vi "calculateSpectraTest.vi"(7 "Reset?":bool, 8 "ErrorIn":errorcluster, 9 "AnalysisSettings":T1={"Fault Thresholds"={"Parameters labels"=[], "Parameters thresholds"=[], "Freqs and thresholds"=[], "Orders and thresholds"=[]}, "Analysis series name"="Analiza", "Save data analysis?"=TRUE, "F-Band Size"=20, "OrderAnalysis?"=TRUE, "Accelerometer"=enum."MMA7351", "fs [Hz]"=4000.0, "Pulse per revolution"=1, "FFT-Parameters"={"averaging mode"=enum."No averaging", "weighting mode"=enum."Linear", "number of averages"=0}, "O-WindowPowerSpectrum"=0, "O-SpectrumAveraging"=enum."No averaging", "O-MaxOrder"=0.0, "O-Resolution"=0.0, "O-BandSize"=0.0, "FrameLength [s]"=1.0, "Aq.FrameLength [ms]"=0, "FilterOrder"=0, "Sensitivity [V/g]"=[]}, 10 "Tacho signal In":waveform(dbl), 11 "AccelerationDataIn":waveform(dbl)[](array[waveform])) -> (0 "ErrorOut":errorcluster, 1 "Rotational speed [RPM]":dbl format="%0.2f", 2 "AccelerationDataFrames":T12, 3 "Tacho signal out":waveform(dbl), 4 "order power spectra":T11(array[cluster]) {"order 0" format="%.2p"; "delta order" format="%.2p"; "magnitude" format="%.2f"}, 5 "AccelerationDataOut":waveform(dbl)[](array[waveform]), 6 "spectrum info":T5[](array[typedef]) {"x-axis units" items=["Time (s)"=0, "Frequency-CB (Hz)"=1, "Frequency-CPB (Hz)"=1248, "Frequency-Arbitrary (Hz)"=2357, "Quefrency (s)"=2, "Revolutions (rev)"=3, "Order"=4, "Speed (RPM)"=11, "Speed (rad/s)"=21, "Index"=65535]; "weighting filter" items=["Linear", "A-weighting", "B-weighting", "C-weighting", "ITU-R 468-4", "Dolby", "CCITT", "C-message", "Wb", "Wc", "Wd", "We", "Wf", "Wh", "Wj", "Wk", "Wm", "AES17 20 kHz lowpass", "AES17 40 kHz lowpass", "AES17 20 kHz highpass", "AES17 40 kHz highpass"]; "dB reference [EU]" format="%.2f"; "engineering units" items=["custom..."=0, "V"=1, "A"=21, "C"=30, "pC"=31, "s"=32, "-"=29, "Pa"=2, "N"=20, "g"=3, "m/s^2"=4, "m/s"=5, "m"=6, "mm/s"=12, "mm"=13, "micron/s"=14, "micron"=15, "in/s^2"=7, "in/s"=8, "in"=9, "mil/s"=10, "mil"=11, "rad/s^2"=16, "rad/s"=17, "rad"=18, "deg/s^2"=26, "deg/s"=27, "deg"=28, "RPM"=22, "cycle/s^2"=23, "Hz"=24, "cycle"=25, "strain"=19]; "spectral info"."window" items=["None "=0, "Hanning"=1, "Hamming"=2, "Blackman-Harris"=3, "Exact Blackman"=4, "Blackman"=5, "Flat Top"=6, "4 Term B-Harris "=7, "7 Term B-Harris"=8, "Low Sidelobe"=9, "Force - Exponential"=10, "Gaussian"=62]})   [LabVIEW 2019]
uses:
  MobileAnalyzer/mainVIs/analyzeAccelerationDataVIs/AccelerationDataFrames.ctl
  <vilib>/addons/_NISVFA/_Shared subVIs/Controls/svc_Spectrum Info.ctl
  <vilib>/addons/_NISVFA/_Shared subVIs/Controls/svc_X-Axis Units.ctl
  <vilib>/addons/_NISVFA/_Shared subVIs/Controls/svc_Spectrum Type.ctl
  <vilib>/addons/_NISVFA/_Shared subVIs/Controls/svc_Engineering Units Text Ring.ctl
  <vilib>/addons/_NISVFA/_Shared subVIs/Controls/svc_Weighting Filter Text Ring.ctl
  <vilib>/addons/_NISVFA/_Shared subVIs/Controls/svc_Complimentary Spectrum Units.ctl
  VibrationDiagnosisDesktopApp/mainVIs/DialogsVIs/AnalysisSettings.ctl
  MobileAnalyzer/mainVIs/analyzeAccelerationDataVIs/calculateFaultIndicatorsVIs/Thresholds.ctl
  MobileAnalyzer/mainVIs/analyzeAccelerationDataVIs/calculateFaultIndicatorsVIs/FaultParameter.ctl
  MobileAnalyzer/mainVIs/aquireAccelerationDataVIs/Accelerometer.ctl
  <vilib>/Analysis/baseanly.llb/Mean (DBL).vi
  <vilib>/measure/maspectr.llb/FFT Spectrum (Mag-Phase) for N Chan.vi
  <vilib>/addons/Sound and Vibration/Order Analysis/Tach Process/OAT Analog Tacho Process (1 Tacho).vi
  <vilib>/addons/Sound and Vibration/Order Analysis/Resample Order Tracking/OAT Convert to Even Angle Signal (N Channels).vi
  <vilib>/addons/Sound and Vibration/Order Analysis/Utility/OAT Output Triggered Even Angle Signal (N Channels).vi
  <vilib>/addons/Sound and Vibration/Order Analysis/Resample Order Tracking/OAT Order Power Spectrum (N Channels).vi
  <vilib>/addons/Sound and Vibration/Order Analysis/Tach Process/SoundVib_TachProcess.lvlib
  <vilib>/addons/Sound and Vibration/Order Analysis/Resample Order Tracking/SoundVib_OrderTracking.lvlib
  <vilib>/Waveform/WDTOps.llb/WDT Waveform Duration DBL.vi
  <vilib>/Waveform/WDTOps.llb/WDT Get Waveform Subset DBL.vi
  <vilib>/Analysis/NI_AALBase.lvlib
  <vilib>/measure/NI_MAPro.lvlib
  <vilib>/addons/Sound and Vibration/Order Analysis/Utility/SoundVib_OAUtility.lvlib
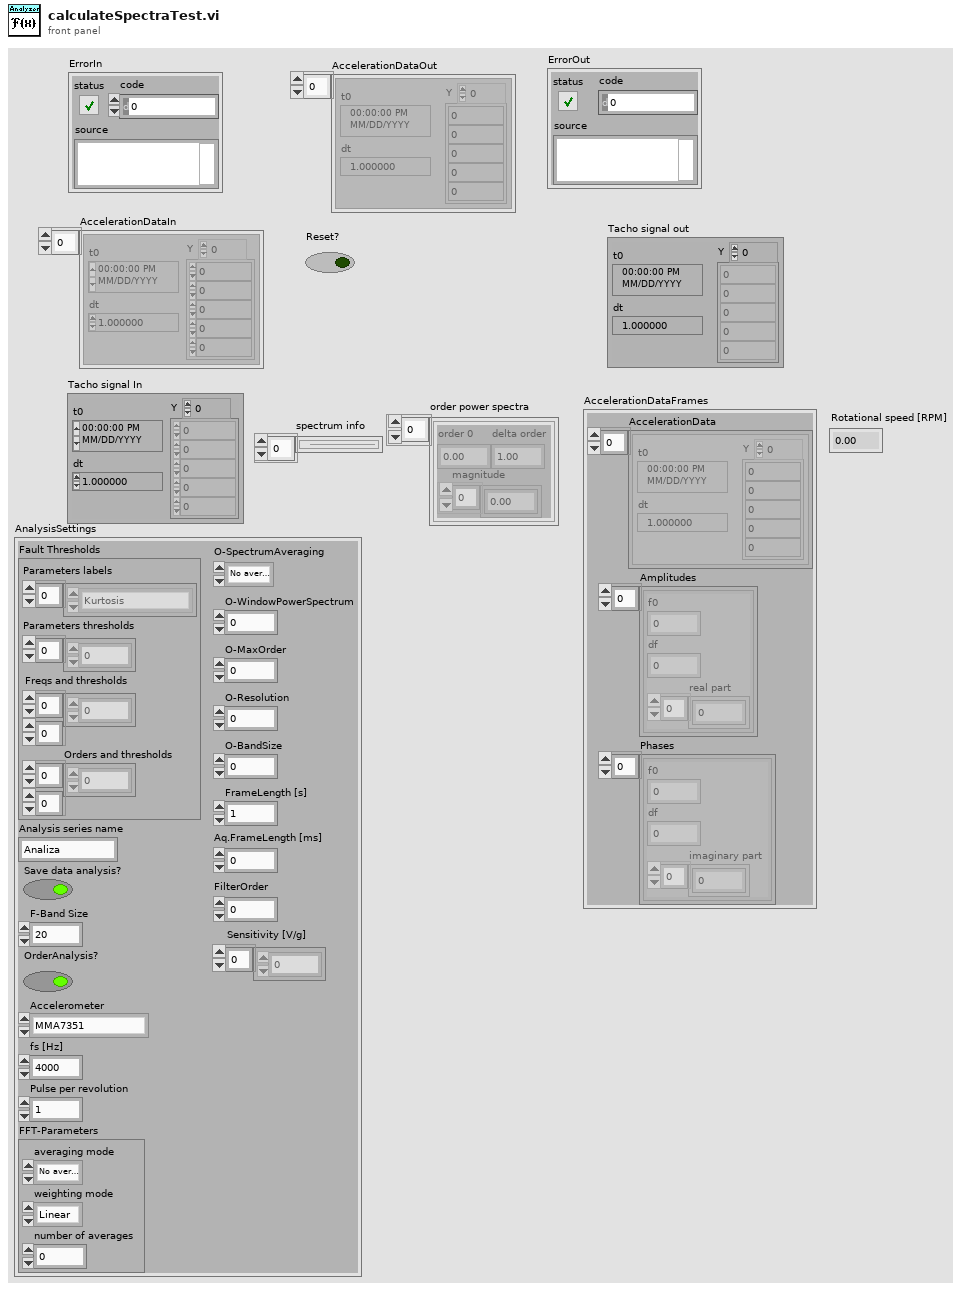
[diagram p1: front panel]
types:
  T1 = typedef "AnalysisSettings.ctl" = cluster{"Fault Thresholds":T2, "Analysis series name":string, "Save data analysis?":bool, "F-Band Size":i32, "OrderAnalysis?":bool, "Accelerometer":T4, "fs [Hz]":dbl, "Pulse per revolution":u16, "FFT-Parameters":cluster{"averaging mode":enum16{"No averaging", "Vector averaging", "RMS averaging", "Peak hold"}, "weighting mode":enum16{"Linear", "Exponential"}, "number of averages":u32}, "O-WindowPowerSpectrum":u32, "O-SpectrumAveraging":enum16{"No averaging", "Vector averaging", "RMS averaging", "Peak hold"}, "O-MaxOrder":dbl, "O-Resolution":dbl, "O-BandSize":dbl, "FrameLength [s]":dbl, "Aq.FrameLength [ms]":i64, "FilterOrder":i32, "Sensitivity [V/g]":dbl[]}
  T2 = typedef "Thresholds.ctl" = cluster{"Parameters labels":T3[], "Parameters thresholds":dbl[], "Freqs and thresholds":dbl[][], "Orders and thresholds":dbl[][]}
  T3 = typedef "FaultParameter.ctl" = enum16{"Kurtosis", "RMS", "Crest factor"}
  T4 = typedef "Accelerometer.ctl" = enum16{"None", "MPU6050", "MMA7351"}
  T5 = typedef "svc_Spectrum Info.ctl" = cluster{"channel name":string, "description":string, "x-axis units":T6, "spectral info":cluster{"spectrum type":T7, "linear/dB":enum16{"linear", "dB"}, "window":u16, "window size":i32, "FFT size":i32}, "engineering units":T8, "custom label":string, "dB reference [EU]":dbl, "peak units":enum16{"rms", "peak", "peak-peak"}, "weighting filter":T9, "spectral density?":bool, "unit label":string, "spectrum skewed?":bool, "complimentary spectrum units":T10}
  T6 = typedef "svc_X-Axis Units.ctl" = u16
  T7 = typedef "svc_Spectrum Type.ctl" = enum16{"FFT Spectrum [complex]", "Amplitude [Magnitude]", "Power [Magnitude^2]", "Cross Spectrum [complex]", "Frequency Response [Complex]"}
  T8 = typedef "svc_Engineering Units Text Ring.ctl" = u16
  T9 = typedef "svc_Weighting Filter Text Ring.ctl" = u16
  T10 = typedef "svc_Complimentary Spectrum Units.ctl" = enum16{"none", "radians", "degrees", "cycles", "imaginary"}
  T11 = cluster{"order 0":dbl, "delta order":dbl, "magnitude":dbl[]}[]
  T12 = typedef "AccelerationDataFrames.ctl" = cluster{"AccelerationData":waveform(dbl)[], "Amplitudes":cluster{"f0":dbl, "df":dbl, "real part":dbl[]}[], "Phases":cluster{"f0":dbl, "df":dbl, "imaginary part":dbl[]}[]}
  T13 = cluster{"averaging mode":enum16{"No averaging", "Vector averaging", "RMS averaging", "Peak hold"}, "weighting mode":enum16{"Linear", "Exponential"}, "number of averages":u32, "linear mode":enum16{"One shot", "Auto restart"}}
  T14 = cluster{"averaging mode":enum16{"No averaging", "Vector averaging", "RMS averaging", "Peak hold"}, "weighting mode":enum16{"Linear", "Exponential"}, "number of averages":u32}
  T15 = enum16{"No averaging", "Vector averaging", "RMS averaging", "Peak hold"}
  T16 = typedef "SoundVib_TachProcess.lvlib/speed profile.ctl" = cluster{"time [s]":dbl[], "speed [RPM]":dbl[]}
  T17 = typedef "svc_Resampled Channel Info.ctl" = cluster{"channel name":string, "description":string, " channel info":T18}
  T18 = typedef "svc_Channel Info.ctl" = cluster{"sensor sensitivity":dbl, "engineering units":T8, "dB reference":dbl, "custom label":string, "weighting filter":T9, "pregain":dbl}
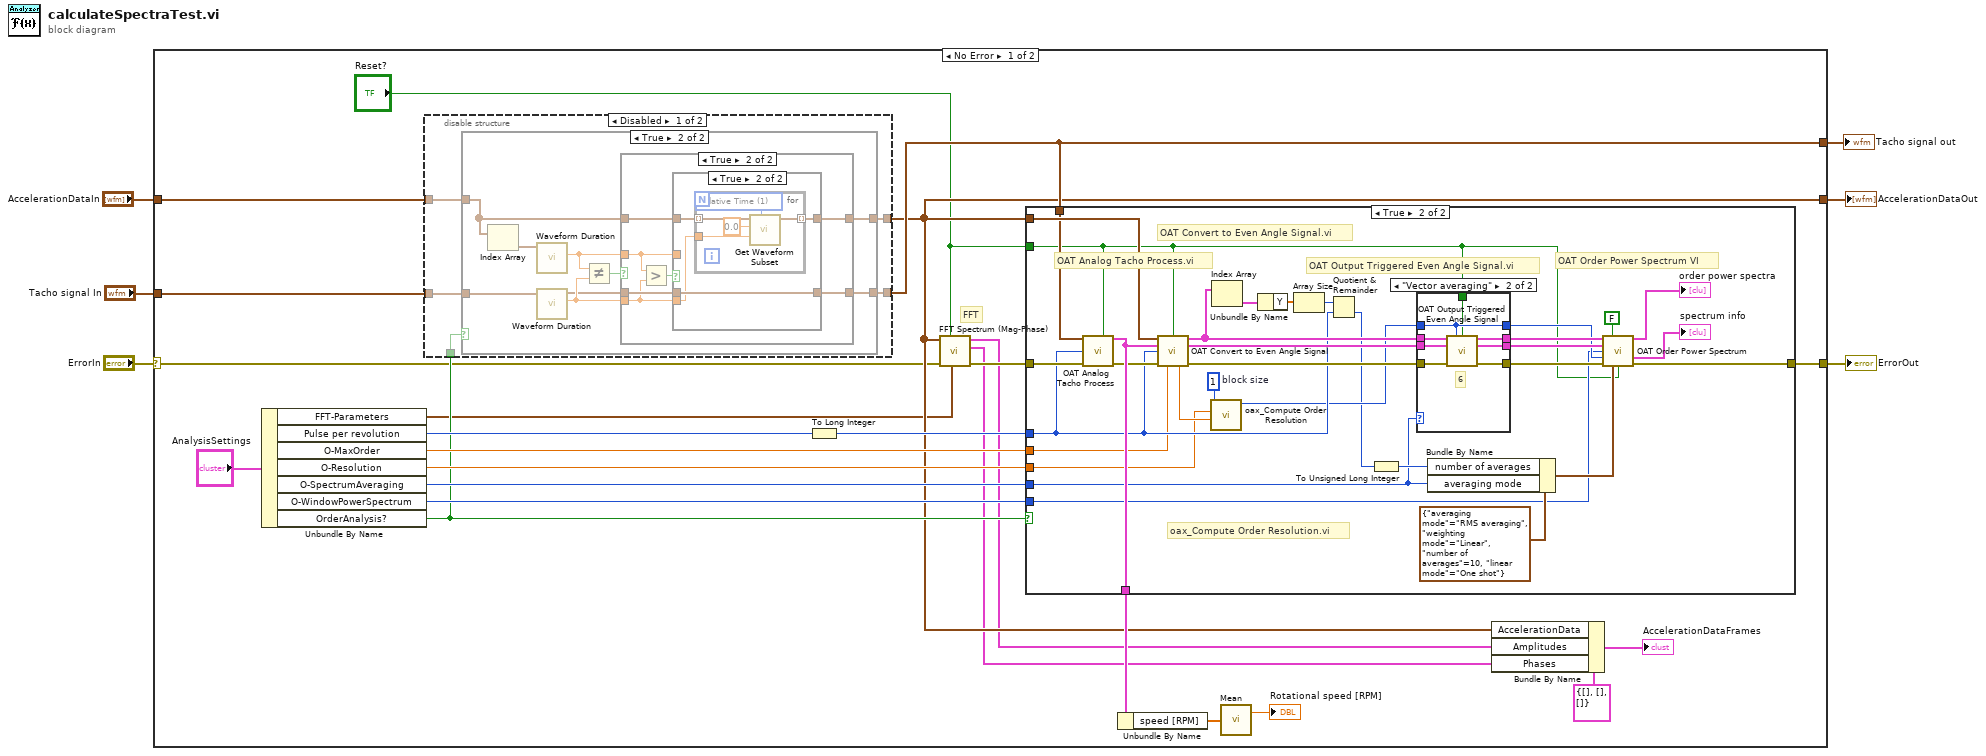
[diagram p0: block diagram]
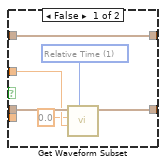
[diagram p4: hidden frame]
diagram:
  n1 = case shown="No Error" "ErrorIn" {
    selector: "ErrorIn" -> [w11 w120]
    tunnel: [w24 w120] -> w6
    tunnel: "AccelerationDataIn" -> [w28 w119]
    tunnel: [w13 w119] -> w3
    tunnel: "Tacho signal In" -> [w27 w118]
    tunnel: [w23 w118] -> w1
    frame No Error {
      # "FFT"
      n2 = Unbundle By Name("AnalysisSettings") -> ("FFT-Parameters"=w10:T14, "Pulse per revolution"=w19:u16, "O-MaxOrder"=w18:dbl, "O-Resolution"=w17:dbl, "O-SpectrumAveraging"=w16:T15, "O-WindowPowerSpectrum"=w15:u32, "OrderAnalysis?"=w14:bool)
      n3 = disable-structure shown="Disabled" {
        disable-tunnel: w28 -> [w35 w72]
        disable-tunnel: w27 -> [w34 w71]
        disable-tunnel: [w33 w71] -> w23
        disable-tunnel: w14 -> [w32 _]
        disable-tunnel: [w31 w72] -> w13
        frame Disabled {
          n4 = case shown="True" w32 {
            tunnel: w35 -> [w37 w41]
            tunnel: w34 -> [w36 w40]
            tunnel: [w37 w39] -> w31
            tunnel: [w36 w38] -> w33
            frame False {
            }
            frame True {
              n5 = Index Array(array=w41) -> (element=w42:waveform(dbl))  [unwired: 1 in]
              n6 = call-poly <vilib>:"Waveform Duration.vi"("waveform in"=w42) -> ("duration"=w45:dbl)  [unwired: 8 in, 2 out]
              n7 = call-poly <vilib>:"Waveform Duration.vi"("waveform in"=w40) -> ("duration"=w46:dbl, "waveform out"=w44:waveform(dbl))  [unwired: 8 in, 1 out]
              n8 = Not Equal?(x=w45, y=w46) -> (x != y?=w43:bool)
              n9 = case shown="True" w43 {
                tunnel: w41 -> [w48 w53]
                tunnel: w44 -> [w47 w54]
                tunnel: [w48 w49] -> w39
                tunnel: [w47 w50] -> w38
                tunnel: w45 -> [_ w52]
                tunnel: w46 -> [_ w51]
                frame False {
                }
                frame True {
                  n10 = Greater?(x=w52, y=w51) -> (0:w55:bool)
                  n11 = case shown="True" w55 {
                    tunnel: w54 -> [w61 w65]
                    tunnel: w53 -> [w58 w64]
                    tunnel: w52 -> [w60 _]
                    tunnel: w51 -> [_ w63]
                    tunnel: [w59 w65] -> w50
                    tunnel: [w58 w62] -> w49
                    frame False {
                      w56 = u16 1 items=["Samples", "Relative Time"] ("start/duration format")
                      n12 = call-poly <vilib>:"Get Waveform Subset.vi"("start/duration format"=w56, "duration"=w60, "start samples/time"=0.0, "waveform in"=w61) -> ("waveform out"=w59:waveform(dbl))  [unwired: 2 in, 3 out]
                    }
                    frame True {
                      n13 = for {
                        tunnel: w64 -> [w70] mode=indexing
                        tunnel: w63 -> [w69]
                        tunnel: [w68] -> w62 mode=indexing
                        w66 = u16 1 items=["Samples", "Relative Time"] ("start/duration format")
                        n14 = call-poly <vilib>:"Get Waveform Subset.vi"("start/duration format"=w66, "duration"=w69, "start samples/time"=0.0, "waveform in"=w70) -> ("waveform out"=w68:waveform(dbl))  [unwired: 2 in, 3 out]
                      }
                    }
                  }
                }
              }
            }
          }
        }
        frame Enabled {
        }
      }
      n15 = To Long Integer(number=w19) -> (32bit integer=w21:i32)
      n16 = call-poly <vilib>:"FFT Spectrum (Mag-Phase).vi"("averaging parameters"=w10, "restart averaging (F)"="Reset?", "error in (no error)"=w11, "time signals"=w13) -> ("error out"=w12:errorcluster, "phases"=w8:cluster{"f0":dbl, "df":dbl, "phase":dbl[]}[], "magnitudes"=w9:cluster{"f0":dbl, "df":dbl, "magnitude":dbl[]}[])  [unwired: 3 in, 2 out]
      n17 = case shown="True" w14 {
        tunnel: w12 -> [w73 w103]
        tunnel: w13 -> [_ w102]
        tunnel: [w73 w101] -> w24
        tunnel: w23 -> [_ w99]
        tunnel: [_ w96] -> w22
        tunnel: w21 -> [_ w88]
        tunnel: w18 -> [_ w78]
        tunnel: w17 -> [_ w77]
        tunnel: w16 -> [_ w76]
        tunnel: w15 -> [_ w75]
        tunnel: "Reset?" -> [_ w74]
        frame False {
        }
        frame True {
          w98 = 1  # block size
          # "oax_Compute Order Resolution.vi"
          # "OAT Order Power Spectrum VI"
          # "OAT Output Triggered Even Angle Signal.vi"
          # "OAT Convert to Even Angle Signal.vi"
          # "OAT Analog Tacho Process.vi"
          n18 = call-poly <vilib>:"OAT Analog Tacho Process.vi"("analog tacho signal"=w99, "reset? (F)"=w74, "pulse/revolution (1)"=w88, "error in (no error)"=w103) -> ("speed profile"=w96:T16, "error out"=w95:errorcluster)  [unwired: 7 in, 3 out]
          n19 = call-poly <vilib>:"OAT Convert to Even Angle Signal.vi"("scaled signals [EU]"=w102, "reset? (F)"=w74, "speed profile"=w96, "pulse/revolution (1)"=w88, "error in (no error)"=w95, "max order (auto)"=w78) -> ("even-angle signals"=w89:cluster{"r0":dbl, "dr":dbl, "Y":dbl[]}[], "even-angle channel info"=w93:T17[], "actual max order"=w97:dbl, "error out"=w94:errorcluster)  [unwired: 5 in, 1 out]
          n20 = call <vilib>:"oax_Compute Order Resolution.vi"("actual max order"=w97, "order resolution"=w77, "block size"=w98) -> ("block size out"=w86:i32)  [unwired: 7 in, 1 out]
          n21 = Index Array(array=w89) -> (element=w92:cluster{"r0":dbl, "dr":dbl, "Y":dbl[]})  [unwired: 1 in]
          n22 = Unbundle By Name(w92) -> ("Y"=w91:dbl[])
          n23 = Array Size(array=w91) -> (size(s)=w90:i32)
          n24 = Quotient & Remainder(x=w90, y=w88) -> (floor(x/y)=w81:i32)  [unwired: 1 out]
          n25 = To Unsigned Long Integer(number=w81) -> (unsigned 32bit integer=w80:u32)
          n26 = case shown="\"Vector averaging\"" w76 {
            tunnel: w94 -> [w108 w117]
            tunnel: [w108 w116] -> w82
            tunnel: w86 -> [w109 w115]
            tunnel: [w109 w115] -> w83
            tunnel: w89 -> [w106 w114]
            tunnel: w93 -> [w107 w113]
            tunnel: [w107 w111] -> w84
            tunnel: [w106 w112] -> w85
            tunnel: w74 -> [_ w110]
            frame "No averaging", Default {
            }
            frame "Vector averaging" {
              # "6"
              n27 = call-poly <vilib>:"OAT Output Triggered Even Angle Signal.vi"("even-angle signals"=w114, "block size"=w115, "reset? (F)"=w110, "even-angle channel info"=w113, "error in (no error)"=w117) -> ("triggered even-angle signals"=w112:cluster{"r0":dbl, "dr":dbl, "Y":dbl[]}[], "even-angle channel info out"=w111:T17[], "error out"=w116:errorcluster)  [unwired: 8 in]
            }
          }
          n28 = Bundle By Name(cluster=T13 {"averaging mode"=enum."RMS averaging", "weighting mode"=enum."Linear", "number of averages"=10, "linear mode"=enum."One shot"} ("averaging parameters"), "number of averages"=w80, "averaging mode"=w76) -> (w79:T13)
          n29 = call-poly <vilib>:"OAT Order Power Spectrum.vi"("even-angle signals"=w85, "dB on? (T)"=FALSE, "even-angle channel info"=w84, "window"=w75, "block size"=w83, "error in (no error)"=w82, "averaging parameters"=w79, "restart averaging? (F)"=w74) -> ("order power spectra"=→"order power spectra":T11, "spectrum info"=→"spectrum info":T5[], "error out"=w101:errorcluster)  [unwired: 1 in, 4 out]
        }
      }
      n30 = Unbundle By Name(w22) -> ("speed [RPM]"=w25:dbl[])
      n31 = call-poly <vilib>:"Mean.vi"("X"=w25) -> ("mean"=→"Rotational speed [RPM]":dbl)  [unwired: 1 out]
      n32 = Bundle By Name(cluster=T12 {"AccelerationData"=[], "Amplitudes"=[], "Phases"=[]} ("AccelerationDataFrames"), "AccelerationData"=w13, "Amplitudes"=w9, "Phases"=w8) -> (→"AccelerationDataFrames":T12)
    }
    frame Error {
    }
  }
  "ErrorOut" <- w6
  "AccelerationDataOut" <- w3
  "Tacho signal out" <- w1
